vi "myRIOXC Update Data.vi"(8 "error in (no error)":errorcluster, 9 "Data In":bool[](array[boolean]), 10 "Facade Ref":refnum<vi>, 11 "Connector Ref":refnum<vi>) -> (0 "error out":errorcluster)   [LabVIEW 2021]
doc: "This VI updates Pin display in xctrl."
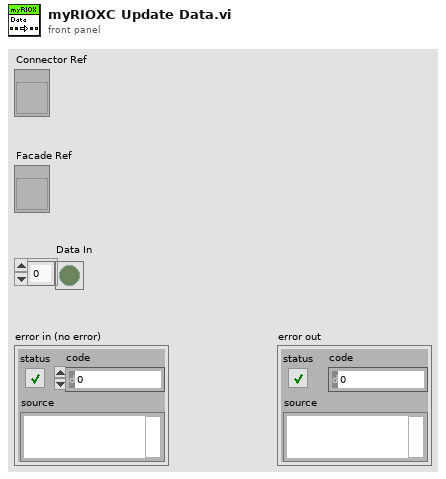
[diagram p1: front panel]
types:
  T1 = enum8{"Enabled", "Disabled", "Disabled and Grayed Out"}
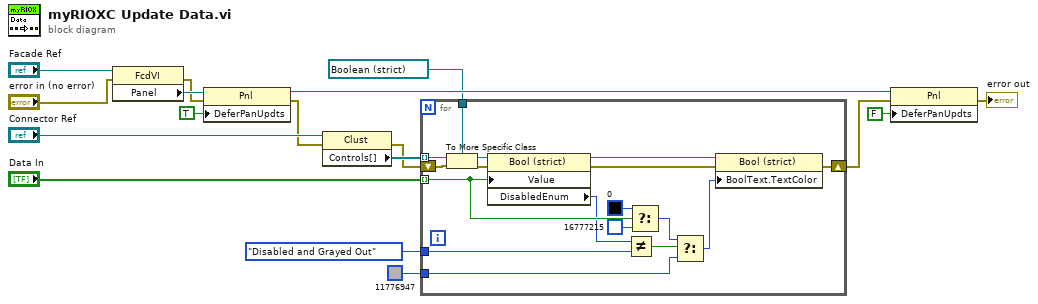
[diagram p0: block diagram]
diagram:
  n1 = property class="FcdVI"(reference="Facade Ref", error in="error in (no error)") -> (error out=w15:errorcluster, "Panel"=w16:refnum<vi>)  [unwired: 1 out]
  n2 = property class="Pnl"(reference=w16, error in=w15, "DeferPanUpdts"=TRUE ("Defer Panel Updates")) -> (reference out=w11:refnum<vi>, error out=w5:errorcluster)
  n3 = property class="Clust"(reference="Connector Ref", error in=w5) -> (error out=w4:errorcluster, "Controls[]"=w17:refnum<vi>[])  [unwired: 1 out]
  n4 = for {
    tunnel: "Data In" -> [w29] mode=indexing
    tunnel: w17 -> [w21] mode=indexing
    shift-right: [w33] -> w10
    shift-left: w4 -> [w19]
    tunnel: refnum<vi> refnum ("Boolean 2") -> [w22]
    tunnel: T1."Disabled and Grayed Out" ("Disabled") -> [w28]
    tunnel: u32 11776947 -> [w24]
    n5 = To More Specific Class(target class=w22, reference=w21, error in=w19) -> (specific class reference=w20:refnum<vi>, error out=w18:errorcluster)
    n6 = property class="Bool (strict)"(reference=w20, error in=w18, "Value"=w29) -> (reference out=w34:refnum<vi>, error out=w32:errorcluster, "DisabledEnum"=w27:T1)
    n7 = Not Equal?(x=w27, y=w28) -> (x != y?=w25:bool)
    n8 = Select(t=u32 0, s=w29, f=u32 16777215) -> (s? t:f=w26:u32)
    n9 = Select(t=w26, s=w25, f=w24) -> (s? t:f=w23:u32)
    n10 = property class="Bool (strict)"(reference=w34, error in=w32, "BoolText.TextColor"=w23) -> (error out=w33:errorcluster)  [unwired: 1 out]
  }
  n11 = property class="Pnl"(reference=w11, error in=w10, "DeferPanUpdts"=FALSE ("Defer Panel Updates")) -> (error out=→"error out":errorcluster)  [unwired: 1 out]
